vi "Simple PID via Cryocon.vi"() -> ()   [LabVIEW 2016]
uses:
  <vilib>/addons/control/pid/pid.llb/PID (DBL).vi
  <vilib>/addons/control/pid/NI_PID_pid.lvlib
panel:
  in  "milliseconds to wait":u32=500
  out "resulting string":string
  out "VISA Resource Name Out":refnum<visa-resource-name>
  out "error out":errorcluster
  in  "error in (no error)":errorcluster
  in  "CryoCon":refnum<visa-resource-name>
  in  "Stop":bool
  out "Process variable and Setpoint":cluster{"initial PV":dbl, "SP:":dbl}(graph)
  in  "PID gains":T1={"proportional gain (Kc)"=2.0, "integral time (Ti, min)"=2.0, "derivative time (Td, min)"=0.001} {"derivative time (Td, min)" format="%.3f"; "integral time (Ti, min)" format="%.3f"; "proportional gain (Kc)" format="%.3f"}
  out "PV:":dbl(slide)=60.754431603254424 scale=0.0..100.0
  in  "SP:":dbl(slide)=43000.0 min=0.0 max=0.0 scale=0.0..100.0
  out "MV:":dbl(slide)=18.78965245852964 scale=-100.0..100.0
  out "Manipulated variable":dbl(graph)
  in  "AH Bridge":refnum<visa-resource-name>
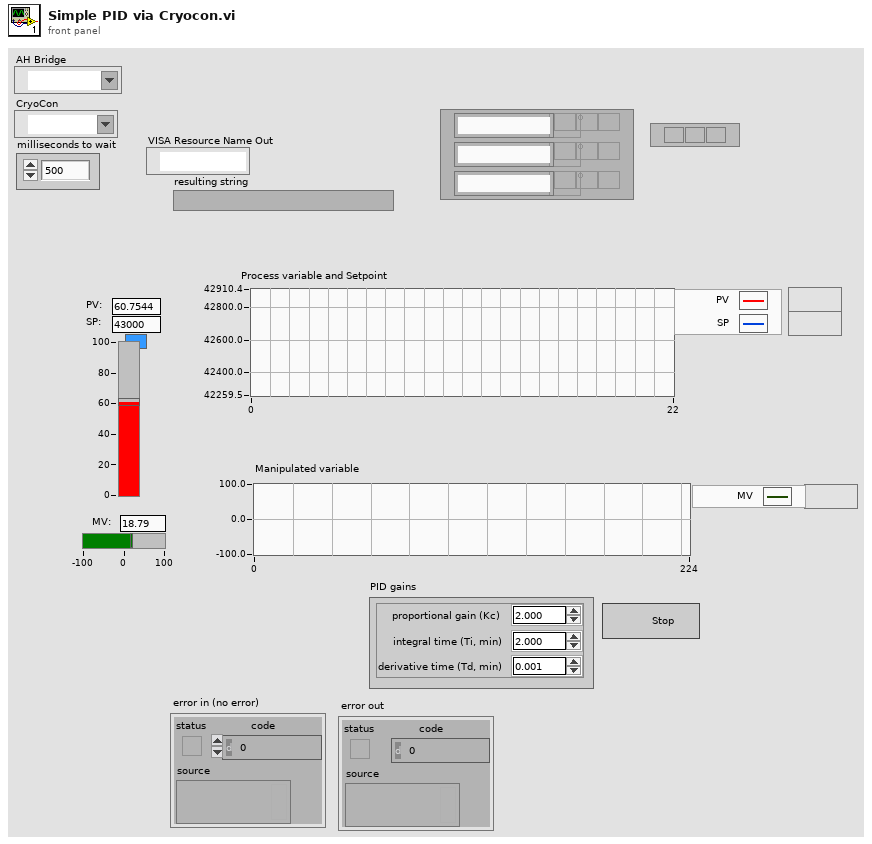
[diagram p1: front panel]
types:
  T1 = cluster{"proportional gain (Kc)":dbl, "integral time (Ti, min)":dbl, "derivative time (Td, min)":dbl}
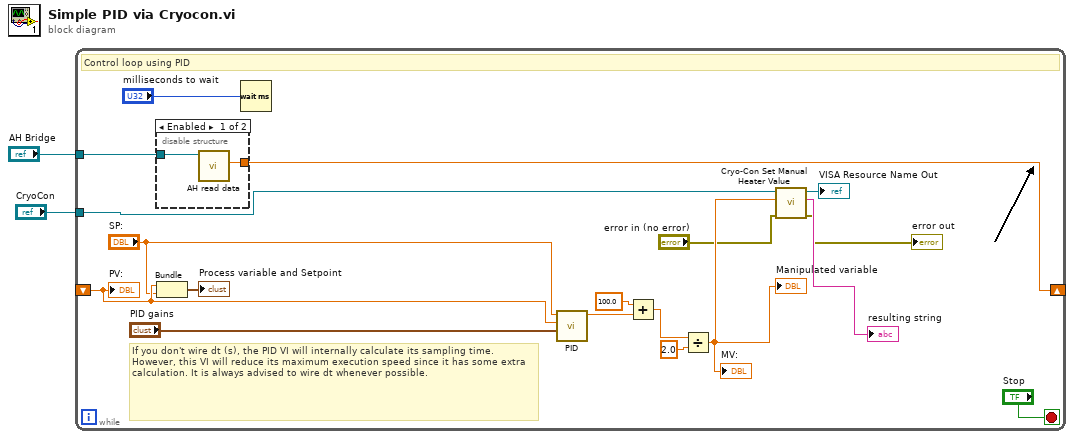
[diagram p0: block diagram]
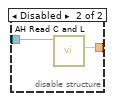
[diagram p2: hidden frame]
diagram:
  n1 = while {
    shift-left: _ -> [w18]
    shift-right: [w15] -> _
    tunnel: "AH Bridge" -> [w14]
    tunnel: "CryoCon" -> [w8]
    stop <- "Stop" stop-if-true
    # "If you don't wire dt (s), the PID VI will internally calculate its sampling time. However, this VI will reduce its maximum execution speed since it has some extra calculation. It is always advised to wire dt whenever possible."
    # "Control loop using PID"
    n2 = disable-structure shown="Enabled" {
      disable-tunnel: [w22 w23] -> w15
      disable-tunnel: w14 -> [w21 w24]
      frame Enabled {
        n3 = call "AH read data.vi"("VISA Resource Name"=w21) -> ("Capacitance"=w22:dbl)  [unwired: 7 in, 3 out]
      }
      frame Disabled {
        n4 = call "AH Read C and L.vi"("VISA resource name"=w24) -> ("Capacitance"=w23:dbl)  [unwired: 7 in, 3 out]
      }
    }
    n5 = Bundle("Capacitance"=w18, "SP:"="SP:") -> (→"Process variable and Setpoint":cluster{"Capacitance":dbl, "SP:":dbl})  [unwired: 1 in]
    n6 = Wait (ms)(milliseconds to wait="milliseconds to wait") -> ()  [unwired: 1 out]
    n7 = call-poly <vilib>:"PID.vi"("PID gains"="PID gains", "process variable"=w18, "setpoint"="SP:") -> ("output"=w12:dbl)  [unwired: 7 in, 1 out]
    n8 = Add(x=100.0, y=w12) -> (x+y=w10:dbl)
    n9 = Divide(x=w10, y=2.0) -> (x/y=w7:dbl)
    "MV:" <- w7
    "Manipulated variable" <- w7
    n10 = call "Cryo-Con Set Manual Heater Value.vi"("error in (no error)"="error in (no error)", "Set heat %"=w7, "VISA Resource Name 2"=w8) -> ("error out"=→"error out":errorcluster, "resulting string"=→"resulting string":string, "VISA Resource Name Out"=→"VISA Resource Name Out":refnum<visa-resource-name>)  [unwired: 6 in]
    "PV:" <- w18
  }
